vi "PSUPanelStore.vi"(8 "Error in":errorcluster, 10 "Experiment State":T1={"error"={"status"=FALSE, "code"=0, "source"=""}, "Digitizer DAQmx Tasks"={"TaskArray"=[]}, "DAQ Settings"={"Channel Settings"=[], "Card Settings"=[]}, "Synchronization Settings"={"Synchronizer 0"="PXI1Slot2", "source terminal"="GlobalSoftwareTrigger", "Synchronizer 1"="PXI1Slot2"}, "DAQ Data"=[], "Next Shot#"="0", "System Message"="", "User Shot Notes"="", "Timing Settings"={"Timing Card Settings"=[], "Timing Channel Settings"=[[{"Delay (s)"=2.559999942779541, "Pulse width (s)"=0.009999999776482582, "Active"=TRUE, "Channel Name"="Fiber 8", "counter"="PXI1Slot8/ctr7", "FrontPanelTime"=2.559999942779541}]]}, "Timing Tasks"={"TaskArray"=[]}, "Tree"="0", "Time Card/Channels"=[2, 8], "DAQ Card/Channels"=[3, 8], "Program Version"="", "RIO Settings"={"Channel Settings"=[], "Card Settings"=[]}, "RIO References"={"Reference Array"=[]}, "RIO Data"={"RIO Deleaved Data"=[], "Raw Readout"=[]}, "RIO Card/Channels"=[3, 8], "DIO Channels"=0, "DIO Settings"={"DIO Channel Array"=[]}, "Global Settings"={"Initial Background Values"={"Reference Shot #"=0.0, "Background pressure [Torr]"=0.0, "Cryo temp [V]"=0.0, "Cryo temp [K]"=0.0, "Cryotemp Calibration File"=path ""}, "Gas Puffing"={"Gas A type"="N", "Gas B type"="N", "Gas C type"="N", "Gas A pressure [psi]"=0.0, "Gas B pressure [psi]"=0.0, "Gas C pressure [psi]"=0.0, "Innner Electrode"="", "Middle Electrode"="", "Outer Electrode"="", "Gas A bottle pressure [psi]"=0.0, "Gas B bottle pressure [psi]"=0.0, "Gas C bottle pressure [psi]"=0.0}, "PSU Voltages"={"Bias1 Voltage [V]"=0.0, "Bias2 Voltage [V]"=0.0, "PSU1 Voltage [V]"=0.0, "Puff-PSU1 CH1 Voltage [V]"=0.0, "Puff-PSU1 CH2 Voltage [V]"=0.0, "Puff-PSU1 CH3 Voltage [V]"=0.0, "PSU2 Voltage [V]"=0.0, "PSU3 Voltage [V]"=0.0}, "TEK 2024B Details"={"CH1"="", "CH2"="", "CH3"="", "CH4"="", "CH1 Ground State"="Grounded", "CH2 Ground State"="Grounded", "CH3 Ground State"="Grounded", "CH4 Ground State"="Grounded"}}, "Calibrations"={"CryoTemp"={"Comment"="", "X"=[], "Y"=[]}, "PSU2 Tach"={"Comment"="", "X"=[], "Y"=[]}, "PSU3 Tach"={"Comment"="", "X"=[], "Y"=[]}, "PSU2 RevTach"={"Comment"="", "X"=[], "Y"=[]}, "PSU3 RevTach"={"Comment"="", "X"=[], "Y"=[]}}, "Tach Tasks"={"PSU2 task"="", "PSU3 task"=""}, "PSU2 Panel Settings"={"PSU2 DIO channels"={"Charge relay DIO"="DAQ0/port0/line3", "Dump relay DIO"="DAQ0/port0/line4", "HV Arm DIO"="DAQ0/port0/line5", "HV On DIO"="DAQ0/port0/line6"}, "PSU2 Tachometer Controls"={"PSU2 Tach Calibration"=path "Z:/Data/Calibration/Tachometer", "PSU2 Charging Voltage [kV]"=0.0, "PSU2 Tach Counter"="DAQ0/port0/line3"}, "PSU2 Reverse Tachometer Controls"={"PSU2 RevTach Calibration"=path "Z:/Data/Calibration/Reverse Tachometer/PSU2_RevTachCalibration.csv", "PSU2 bank Voltage [kV]"=0.0, "PSU2 RevTach Counter"=""}}, "PSU3 Panel Settings"={"PSU3 DIO channels"={"Charge relay DIO"="DAQ0/port0/line5", "Dump relay DIO"="DAQ0/port0/line6", "HV Arm DIO"="", "HV On DIO"="DAQ0/port0/line6"}, "PSU3 Tachometer Controls"={"PSU3 Tach Calibration"=path "Z:/Data/Calibration/Reverse Tachometer/PSU3_RevTachCalibration.csv", "PSU3 Charging Voltage [kV]"=0.0, "PSU3 Tach Counter"=""}, "PSU3 Reverse Tachometer Controls"={"PSU3 RevTach Calibration"=path "Z:/Data/Calibration/Reverse Tachometer/PSU3_RevTachCalibration.csv", "PSU3 bank Voltage [kV]"=0.0, "PSU3 RevTach Counter"=""}}} {"Global Settings"."Initial Background Values"."Cryo temp [K]" format="%#_4g"; "RIO Settings"."Card Settings"."Sample Rate" format="%#_3p"; "Timing Settings"."Timing Channel Settings"."FrontPanelTime" format="%.3p"; "Timing Settings"."Timing Channel Settings"."Pulse width (s)" format="%.3p"; "Timing Settings"."Timing Channel Settings"."Delay (s)" format="%.3p"; "DAQ Settings"."Card Settings"."Global Edge Type" items=["Rising"=10280, "Falling"=10171]; "DAQ Settings"."Card Settings"."Sample Rate" format="%#_3p"}, 11 "Tree DVR In":refnum<data-value>) -> (0 "Error out":errorcluster)   [LabVIEW 2015]
uses:
  Controls/ExperimentStateCluster.ctl
  Controls/DigitizerSettingsChannelSettings.ctl
  Controls/DigitizerSettingsCardSettingsArray.ctl
  Controls/DigitizerSettingsCardSettings.ctl
  Controls/TimingSettings.ctl
  Controls/TimingCardSettings.ctl
  Controls/TimingChannelSettings.ctl
  Controls/RIOSettingsExperimentStateCluster.ctl
  Controls/RIOChannelSettingsArrayExperimentStateCluster.ctl
  Controls/RIOSettingsChannelSettings.ctl
  Controls/RIOSettingsCardSettingsArray.ctl
  Controls/RIOSettingsCardSettings.ctl
  <vilib>/userdefined/High Color/nirio_resource_hc.ctl
  Controls/RIOData.ctl
  Controls/DIOChannel.ctl
  Controls/Global Settings/GlobalSettings.ctl
  Controls/Global Settings/InitialBackgroundValues.ctl
  Controls/Global Settings/GasPuffing.ctl
  Controls/Global Settings/PSUVoltages.ctl
  Controls/Global Settings/ScopeDetails.ctl
  Controls/Calibrations/Calibrations.ctl
  Controls/Calibrations/CryoTemoCalibration.ctl
  Controls/Calibrations/PSU2TachCalibration.ctl
  Controls/Calibrations/PSU3TachCalibration.ctl
  Controls/TachTasks.ctl
  Controls/PSU2PanelSettings.ctl
  Controls/PSU2DIOChannels.ctl
  Controls/PSU2TachometerControls.ctl
  Controls/PSU2ReverseTachometerControls.ctl
  Controls/PSU3PanelSettings.ctl
  Controls/PSU3DIOChannels.ctl
  Controls/PSU3TachometerControls.ctl
  Controls/PSU3ReverseTachometerControls.ctl
  <vilib>/MDSplus/Classes/Tree_Class/Tree.lvclass
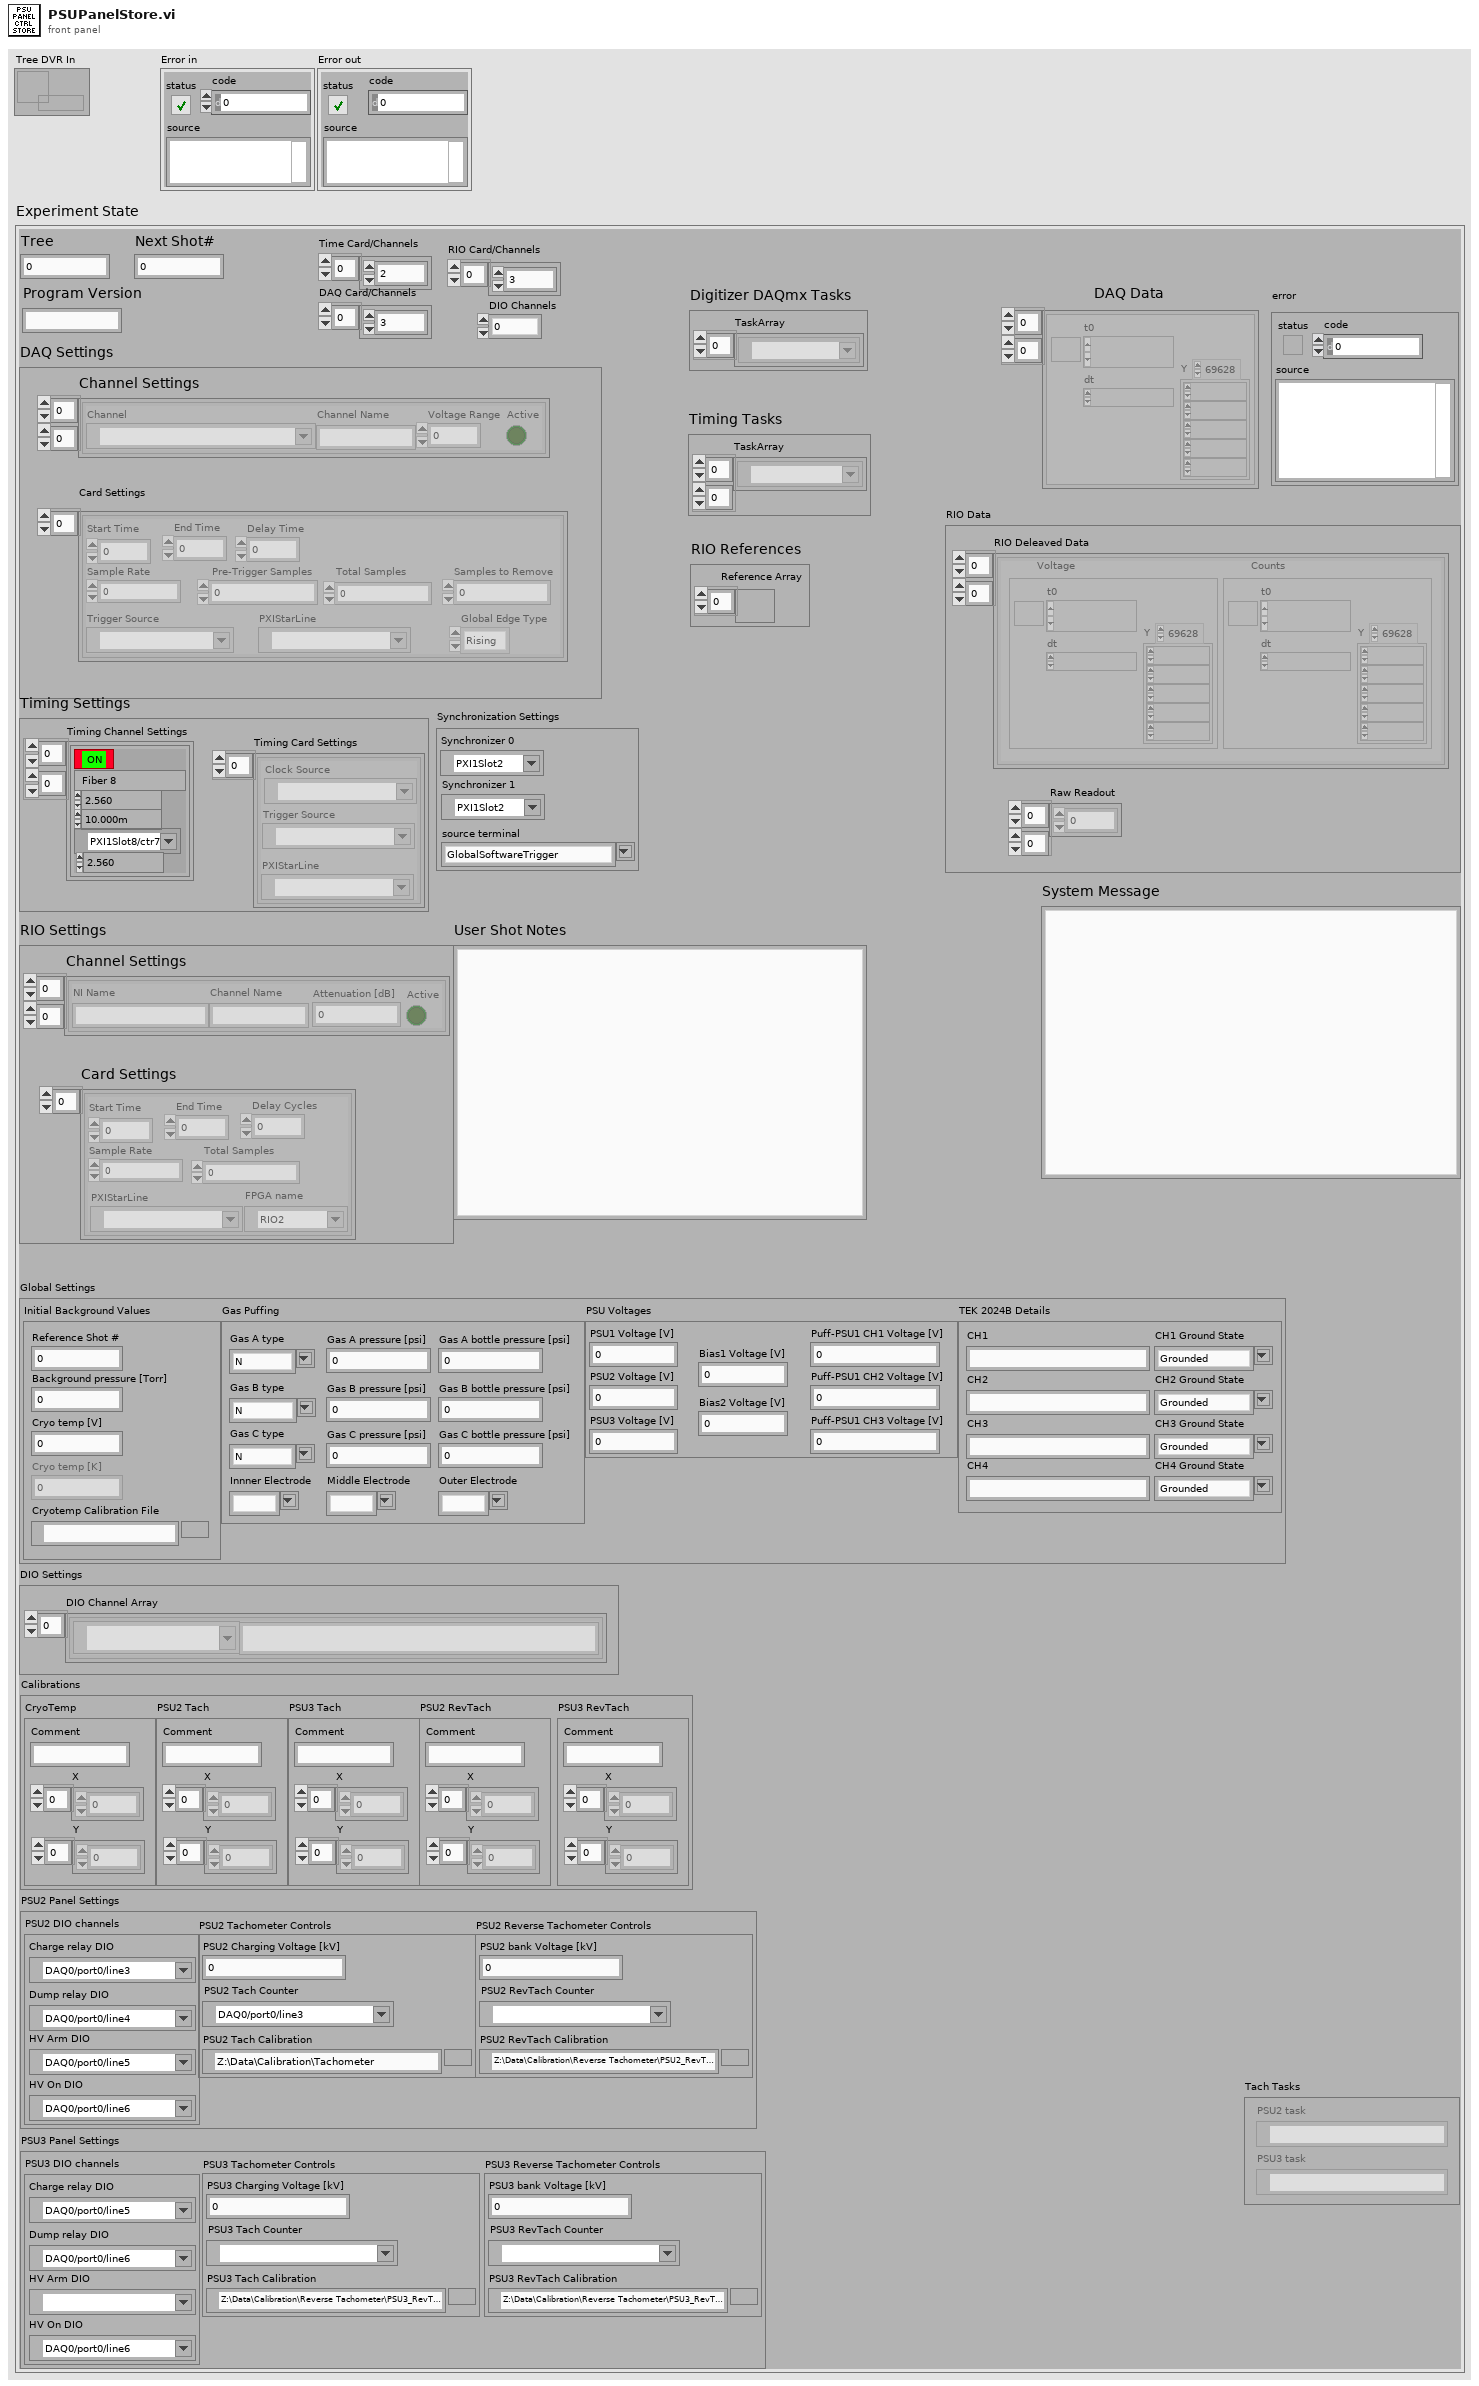
[diagram p1: front panel]
types:
  T1 = typedef "ExperimentStateCluster.ctl" = cluster{"error":errorcluster, "Digitizer DAQmx Tasks":cluster{"TaskArray":refnum<k21>[]}, "DAQ Settings":cluster{"Channel Settings":T2[][], "Card Settings":T3}, "Synchronization Settings":cluster{"Synchronizer 0":refnum<k15>, "source terminal":string, "Synchronizer 1":refnum<k15>}, "DAQ Data":waveform(dbl)[][], "Next Shot#":string, "System Message":string, "User Shot Notes":string, "Timing Settings":T5, "Timing Tasks":cluster{"TaskArray":refnum<k21>[][]}, "Tree":string, "Time Card/Channels":i32[], "DAQ Card/Channels":i32[], "Program Version":string, "RIO Settings":T8, "RIO References":cluster{"Reference Array":refnum<k20>[]}, "RIO Data":T14, "RIO Card/Channels":i32[], "DIO Channels":i32, "DIO Settings":cluster{"DIO Channel Array":T15[]}, "Global Settings":T16, "Calibrations":T21, "Tach Tasks":T25, "PSU2 Panel Settings":T26, "PSU3 Panel Settings":T30}
  T2 = typedef "DigitizerSettingsChannelSettings.ctl" = cluster{"Channel":tag, "Channel Name":string, "Voltage Range":dbl, "Active":bool}
  T3 = typedef "DigitizerSettingsCardSettingsArray.ctl" = T4[]
  T4 = typedef "DigitizerSettingsCardSettings.ctl" = cluster{"Start Time":dbl, "End Time":dbl, "Sample Rate":dbl, " Pre-Trigger Samples":u32, "Total Samples":i32, "Samples to Remove":u32, "Trigger Source":tag, "Global Edge Type":i32, "PXIStarLine":tag, "Delay Time":dbl}
  T5 = typedef "TimingSettings.ctl" = cluster{"Timing Card Settings":T6[], "Timing Channel Settings":T7[][]}
  T6 = typedef "TimingCardSettings.ctl" = cluster{"Trigger Source":tag, "Clock Source":tag, "PXIStarLine":tag}
  T7 = typedef "TimingChannelSettings.ctl" = cluster{"Delay (s)":dbl, "Pulse width (s)":dbl, "Active":bool, "Channel Name":string, "counter":tag, "FrontPanelTime":dbl}
  T8 = typedef "RIOSettingsExperimentStateCluster.ctl" = cluster{"Channel Settings":T9, "Card Settings":T11}
  T9 = typedef "RIOChannelSettingsArrayExperimentStateCluster.ctl" = T10[][]
  T10 = typedef "RIOSettingsChannelSettings.ctl" = cluster{"Channel Name":string, "Active":bool, "NI Name":string, "Attenuation [dB]":i32}
  T11 = typedef "RIOSettingsCardSettingsArray.ctl" = T12[]
  T12 = typedef "RIOSettingsCardSettings.ctl" = cluster{"Start Time":dbl, "End Time":dbl, "Sample Rate":dbl, "Total Samples":u64, "PXIStarLine":tag, "Delay Cycles":u64, "FPGA name":T13}
  T13 = typedef "nirio_resource_hc.ctl" = tag
  T14 = typedef "RIOData.ctl" = cluster{"RIO Deleaved Data":cluster{"Voltage":waveform(dbl), "Counts":waveform(i16)}[][], "Raw Readout":u64[][]}
  T15 = typedef "DIOChannel.ctl" = cluster{"Channel Name":string, "NI Name":tag}
  T16 = typedef "GlobalSettings.ctl" = cluster{"Initial Background Values":T17, "Gas Puffing":T18, "PSU Voltages":T19, "TEK 2024B Details":T20}
  T17 = typedef "InitialBackgroundValues.ctl" = cluster{"Reference Shot #":dbl, "Background pressure [Torr]":dbl, "Cryo temp [V]":dbl, "Cryo temp [K]":dbl, "Cryotemp Calibration File":path}
  T18 = typedef "GasPuffing.ctl" = cluster{"Gas A type":string, "Gas B type":string, "Gas C type":string, "Gas A pressure [psi]":dbl, "Gas B pressure [psi]":dbl, "Gas C pressure [psi]":dbl, "Innner Electrode":string, "Middle Electrode":string, "Outer Electrode":string, "Gas A bottle pressure [psi]":dbl, "Gas B bottle pressure [psi]":dbl, "Gas C bottle pressure [psi]":dbl}
  T19 = typedef "PSUVoltages.ctl" = cluster{"Bias1 Voltage [V]":dbl, "Bias2 Voltage [V]":dbl, "PSU1 Voltage [V]":dbl, "Puff-PSU1 CH1 Voltage [V]":dbl, "Puff-PSU1 CH2 Voltage [V]":dbl, "Puff-PSU1 CH3 Voltage [V]":dbl, "PSU2 Voltage [V]":dbl, "PSU3 Voltage [V]":dbl}
  T20 = typedef "ScopeDetails.ctl" = cluster{"CH1":string, "CH2":string, "CH3":string, "CH4":string, "CH1 Ground State":string, "CH2 Ground State":string, "CH3 Ground State":string, "CH4 Ground State":string}
  T21 = typedef "Calibrations.ctl" = cluster{"CryoTemp":T22, "PSU2 Tach":T23, "PSU3 Tach":T24, "PSU2 RevTach":T23, "PSU3 RevTach":T24}
  T22 = typedef "CryoTemoCalibration.ctl" = cluster{"Comment":string, "X":dbl[], "Y":dbl[]}
  T23 = typedef "PSU2TachCalibration.ctl" = cluster{"Comment":string, "X":dbl[], "Y":dbl[]}
  T24 = typedef "PSU3TachCalibration.ctl" = cluster{"Comment":string, "X":dbl[], "Y":dbl[]}
  T25 = typedef "TachTasks.ctl" = cluster{"PSU2 task":refnum<k21>, "PSU3 task":refnum<k21>}
  T26 = typedef "PSU2PanelSettings.ctl" = cluster{"PSU2 DIO channels":T27, "PSU2 Tachometer Controls":T28, "PSU2 Reverse Tachometer Controls":T29}
  T27 = typedef "PSU2DIOChannels.ctl" = cluster{"Charge relay DIO":tag, "Dump relay DIO":tag, "HV Arm DIO":tag, "HV On DIO":tag}
  T28 = typedef "PSU2TachometerControls.ctl" = cluster{"PSU2 Tach Calibration":path, "PSU2 Charging Voltage [kV]":dbl, "PSU2 Tach Counter":tag}
  T29 = typedef "PSU2ReverseTachometerControls.ctl" = cluster{"PSU2 RevTach Calibration":path, "PSU2 bank Voltage [kV]":dbl, "PSU2 RevTach Counter":tag}
  T30 = typedef "PSU3PanelSettings.ctl" = cluster{"PSU3 DIO channels":T31, "PSU3 Tachometer Controls":T32, "PSU3 Reverse Tachometer Controls":T33}
  T31 = typedef "PSU3DIOChannels.ctl" = cluster{"Charge relay DIO":tag, "Dump relay DIO":tag, "HV Arm DIO":tag, "HV On DIO":tag}
  T32 = typedef "PSU3TachometerControls.ctl" = cluster{"PSU3 Tach Calibration":path, "PSU3 Charging Voltage [kV]":dbl, "PSU3 Tach Counter":tag}
  T33 = typedef "PSU3ReverseTachometerControls.ctl" = cluster{"PSU3 RevTach Calibration":path, "PSU3 bank Voltage [kV]":dbl, "PSU3 RevTach Counter":tag}
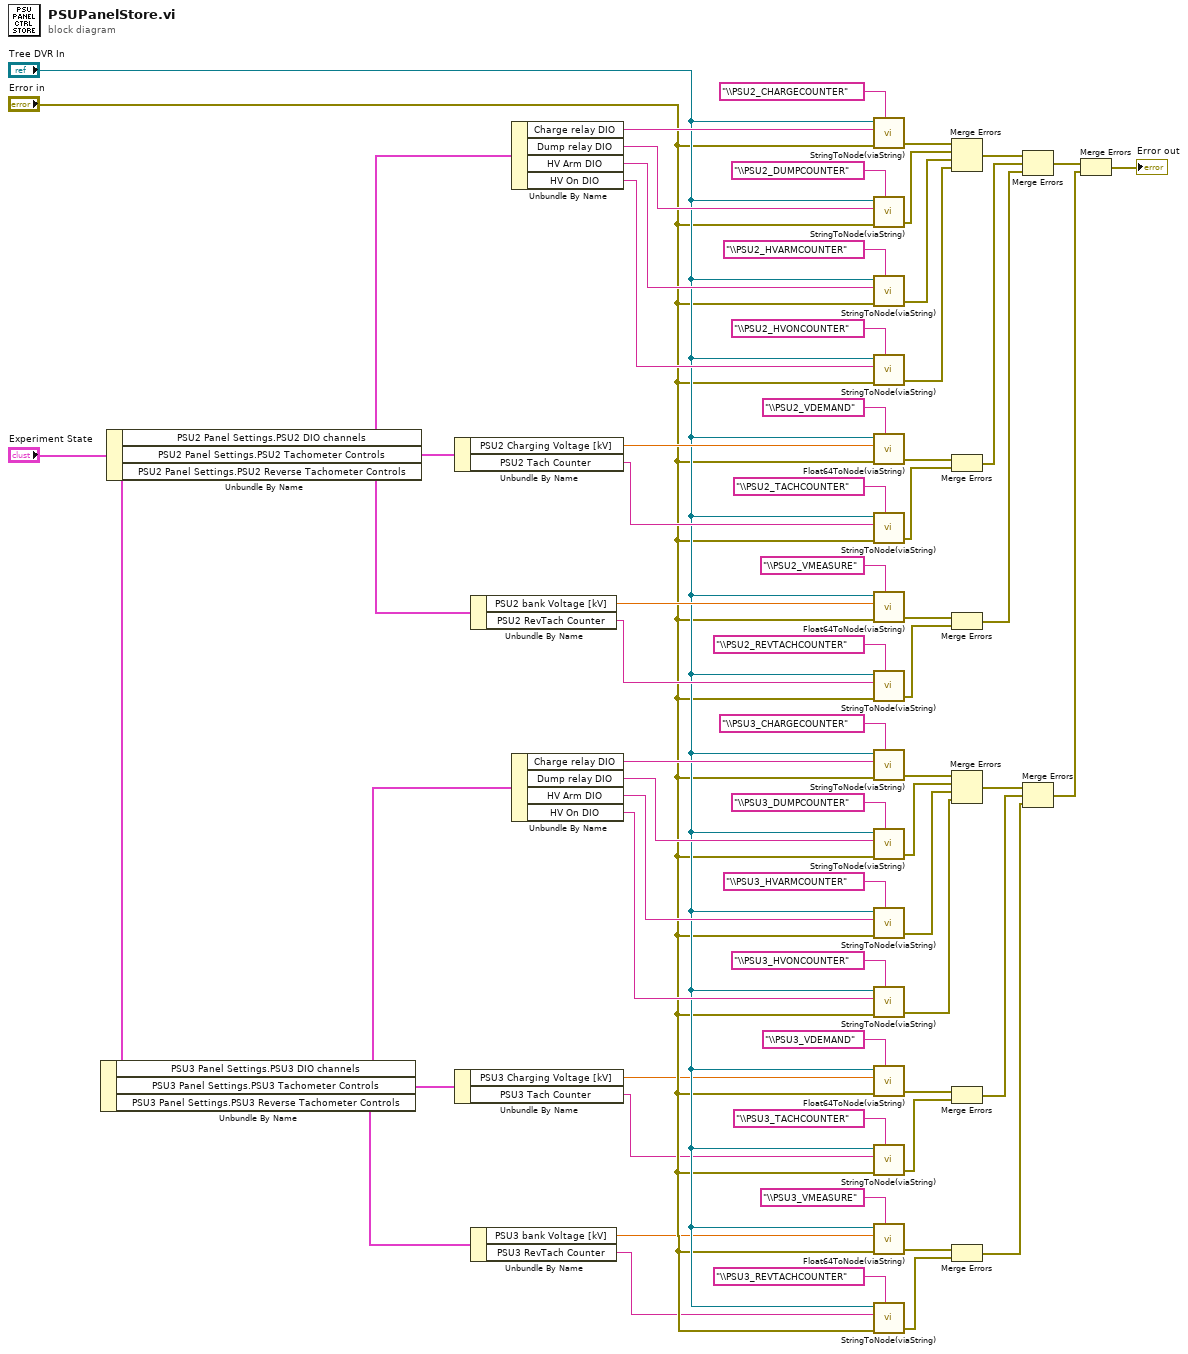
[diagram p0: block diagram]
diagram:
  n1 = Unbundle By Name("Experiment State") -> ("PSU3 Panel Settings.PSU3 DIO channels"=w59:T31, "PSU3 Panel Settings.PSU3 Tachometer Controls"=w58:T32, "PSU3 Panel Settings.PSU3 Reverse Tachometer Controls"=w57:T33)
  n2 = Unbundle By Name("Experiment State") -> ("PSU2 Panel Settings.PSU2 DIO channels"=w62:T27, "PSU2 Panel Settings.PSU2 Tachometer Controls"=w61:T28, "PSU2 Panel Settings.PSU2 Reverse Tachometer Controls"=w60:T29)
  n3 = Unbundle By Name(w61) -> ("PSU2 Charging Voltage [kV]"=w34:dbl, "PSU2 Tach Counter"=w33:tag)
  n4 = Unbundle By Name(w58) -> ("PSU3 Charging Voltage [kV]"=w4:dbl, "PSU3 Tach Counter"=w3:tag)
  n5 = Unbundle By Name(w60) -> ("PSU2 bank Voltage [kV]"=w30:dbl, "PSU2 RevTach Counter"=w29:tag)
  n6 = Unbundle By Name(w57) -> ("PSU3 bank Voltage [kV]"=w2:dbl, "PSU3 RevTach Counter"=w1:tag)
  n7 = Unbundle By Name(w62) -> ("Charge relay DIO"=w45:tag, "Dump relay DIO"=w44:tag, "HV Arm DIO"=w43:tag, "HV On DIO"=w42:tag)
  n8 = Unbundle By Name(w59) -> ("Charge relay DIO"=w18:tag, "Dump relay DIO"=w17:tag, "HV Arm DIO"=w16:tag, "HV On DIO"=w15:tag)
  n9 = call "StringToNode(viaString).vi"("Tree DVR in"="Tree DVR In", "String value in"=w45, "error in (no error)"="Error in", "NodePath"="\\PSU2_CHARGECOUNTER") -> ("error out"=w49:errorcluster)  [unwired: 3 in]
  n10 = call "StringToNode(viaString).vi"("Tree DVR in"="Tree DVR In", "String value in"=w44, "error in (no error)"="Error in", "NodePath"="\\PSU2_DUMPCOUNTER") -> ("error out"=w41:errorcluster)  [unwired: 3 in]
  n11 = call "StringToNode(viaString).vi"("Tree DVR in"="Tree DVR In", "String value in"=w43, "error in (no error)"="Error in", "NodePath"="\\PSU2_HVARMCOUNTER") -> ("error out"=w40:errorcluster)  [unwired: 3 in]
  n12 = call "StringToNode(viaString).vi"("Tree DVR in"="Tree DVR In", "String value in"=w42, "error in (no error)"="Error in", "NodePath"="\\PSU2_HVONCOUNTER") -> ("error out"=w39:errorcluster)  [unwired: 3 in]
  n13 = call "Float64ToNode(viaString).vi"("Tree DVR in"="Tree DVR In", "DBL in"=w34, "error in"="Error in", "NodePath"="\\PSU2_VDEMAND") -> ("error out"=w36:errorcluster)  [unwired: 3 in]
  n14 = call "StringToNode(viaString).vi"("Tree DVR in"="Tree DVR In", "String value in"=w33, "error in (no error)"="Error in", "NodePath"="\\PSU2_TACHCOUNTER") -> ("error out"=w35:errorcluster)  [unwired: 3 in]
  n15 = call "Float64ToNode(viaString).vi"("Tree DVR in"="Tree DVR In", "DBL in"=w30, "error in"="Error in", "NodePath"="\\PSU2_VMEASURE") -> ("error out"=w28:errorcluster)  [unwired: 3 in]
  n16 = call "StringToNode(viaString).vi"("Tree DVR in"="Tree DVR In", "String value in"=w29, "error in (no error)"="Error in", "NodePath"="\\PSU2_REVTACHCOUNTER") -> ("error out"=w27:errorcluster)  [unwired: 3 in]
  n17 = call "StringToNode(viaString).vi"("Tree DVR in"="Tree DVR In", "String value in"=w18, "error in (no error)"="Error in", "NodePath"="\\PSU3_CHARGECOUNTER") -> ("error out"=w12:errorcluster)  [unwired: 3 in]
  n18 = call "StringToNode(viaString).vi"("Tree DVR in"="Tree DVR In", "String value in"=w17, "error in (no error)"="Error in", "NodePath"="\\PSU3_DUMPCOUNTER") -> ("error out"=w11:errorcluster)  [unwired: 3 in]
  n19 = call "StringToNode(viaString).vi"("Tree DVR in"="Tree DVR In", "String value in"=w16, "error in (no error)"="Error in", "NodePath"="\\PSU3_HVARMCOUNTER") -> ("error out"=w10:errorcluster)  [unwired: 3 in]
  n20 = call "StringToNode(viaString).vi"("Tree DVR in"="Tree DVR In", "String value in"=w15, "error in (no error)"="Error in", "NodePath"="\\PSU3_HVONCOUNTER") -> ("error out"=w9:errorcluster)  [unwired: 3 in]
  n21 = call "Float64ToNode(viaString).vi"("Tree DVR in"="Tree DVR In", "DBL in"=w4, "error in"="Error in", "NodePath"="\\PSU3_VDEMAND") -> ("error out"=w8:errorcluster)  [unwired: 3 in]
  n22 = call "StringToNode(viaString).vi"("Tree DVR in"="Tree DVR In", "String value in"=w3, "error in (no error)"="Error in", "NodePath"="\\PSU3_TACHCOUNTER") -> ("error out"=w7:errorcluster)  [unwired: 3 in]
  n23 = call "Float64ToNode(viaString).vi"("Tree DVR in"="Tree DVR In", "DBL in"=w2, "error in"="Error in", "NodePath"="\\PSU3_VMEASURE") -> ("error out"=w6:errorcluster)  [unwired: 3 in]
  n24 = call "StringToNode(viaString).vi"("Tree DVR in"="Tree DVR In", "String value in"=w1, "error in (no error)"="Error in", "NodePath"="\\PSU3_REVTACHCOUNTER") -> ("error out"=w5:errorcluster)  [unwired: 3 in]
  n25 = Merge Errors(w49, w41, w40, w39) -> (w66:errorcluster)
  n26 = Merge Errors(w36, w35) -> (w65:errorcluster)
  n27 = Merge Errors(w28, w27) -> (w64:errorcluster)
  n28 = Merge Errors(w12, w11, w10, w9) -> (w52:errorcluster)
  n29 = Merge Errors(w8, w7) -> (w53:errorcluster)
  n30 = Merge Errors(w6, w5) -> (w54:errorcluster)
  n31 = Merge Errors(w66, w65, w64) -> (w56:errorcluster)
  n32 = Merge Errors(w52, w53, w54) -> (w51:errorcluster)
  n33 = Merge Errors(w56, w51) -> (→"Error out":errorcluster)
